vi "InitAE-Groups.vi"(8 "Error In":errorcluster, 11 "LstBox Refnum":refnum<vi>) -> (0 "Error Out":errorcluster)   [LabVIEW 2017, in "Client.lvlib" / "UI_API.lvlib"]
uses:
  UI_API.lvlib
panel:
  in  "AE Group":T1(ring)
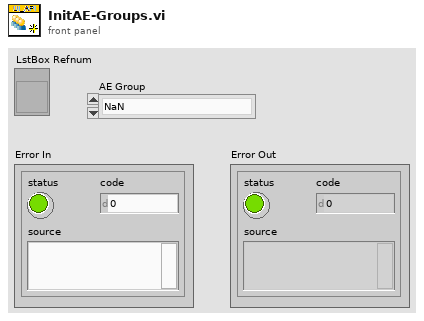
[diagram p1: front panel]
types:
  T1 = enum32{"NaN", "AE-Germany", "AE-Poland", "AE-Switzerland", "AE-Czech Republic", "AE-Hungary", "AE-Romania", "AE-Slovakia", "AE-Slovenia"}
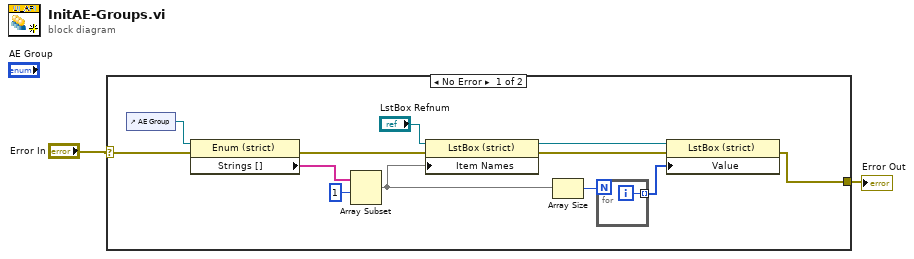
[diagram p0: block diagram]
diagram:
  n1 = case shown="No Error" "Error In" {
    selector: "Error In" -> [w12 w16]
    tunnel: [w6 w16] -> w1
    frame No Error {
      n2 = control-ref of="AE Group"() -> (w14:refnum<vi>)
      n3 = property class="Enum (strict)"(reference=w14, error in=w12) -> (error out=w11:errorcluster, "Strings []"=w10:string[])  [unwired: 1 out]
      n4 = Array Subset(array=w10, index=1) -> (w5:string[])  [unwired: 1 in]
      n5 = property class="LstBox (strict)"(reference="LstBox Refnum", error in=w11, "Item Names"=w5) -> (reference out=w8:refnum<vi>, error out=w7:errorcluster)
      n6 = Array Size(array=w5) -> (size(s)=w4:i32)
      n7 = for {
        N: w4 -> [_]
        tunnel: [w15] -> w3 mode=indexing
        i -> [w15]
      }
      n8 = property class="LstBox (strict)"(reference=w8, error in=w7, "Value"=w3) -> (error out=w6:errorcluster)  [unwired: 1 out]
    }
    frame Error {
    }
  }
  "Error Out" <- w1
